vi "Oscilloscope Type Axis Scale.vi"(8 "Error In":errorcluster, 9 "Volts/Div":dbl, 11 "Graph In":refnum<vi>) -> (0 "Error Out":errorcluster, 3 "Graph Out":refnum<vi>)   [LabVIEW 2017]
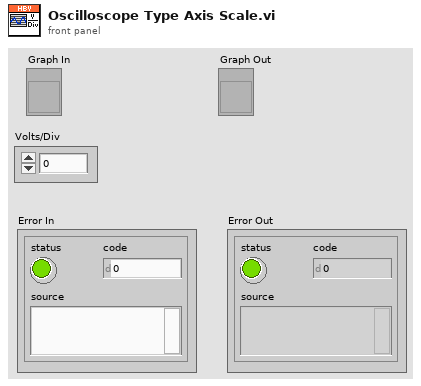
[diagram p1: front panel]
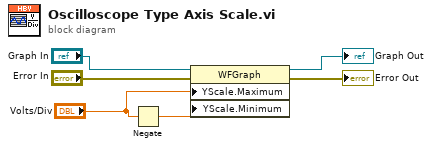
[diagram p0: block diagram]
diagram:
  n1 = Negate(x="Volts/Div") -> (-x=w2:dbl)
  n2 = property on="Property Node" class="WFGraph"(reference="Graph In", error in="Error In", "YScale.Maximum"="Volts/Div", "YScale.Minimum"=w2) -> (reference out=→"Graph Out":refnum<vi>, error out=→"Error Out":errorcluster)
